vi "Fetch.vi"(8 "error in (no error)":errorcluster, 10 "Fetch Type":i32(ring) items=["CURR", "VOLT", "POW"], 11 "VISA resource name":refnum<visa-resource-name>) -> (0 "error out":errorcluster, 2 "Value":dbl, 3 "VISA resource name out":refnum<visa-resource-name>)   [LabVIEW 2020, in "IT6500.lvlib"]
doc: "<b>Valid Values:</b>\n0:Get Current\n1:Get Voltage\n2:Get Power\n\nDefault: 0:Get Current"
uses:
  IT6500.lvlib
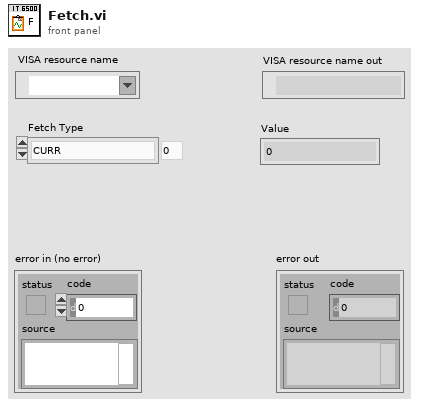
[diagram p1: front panel]
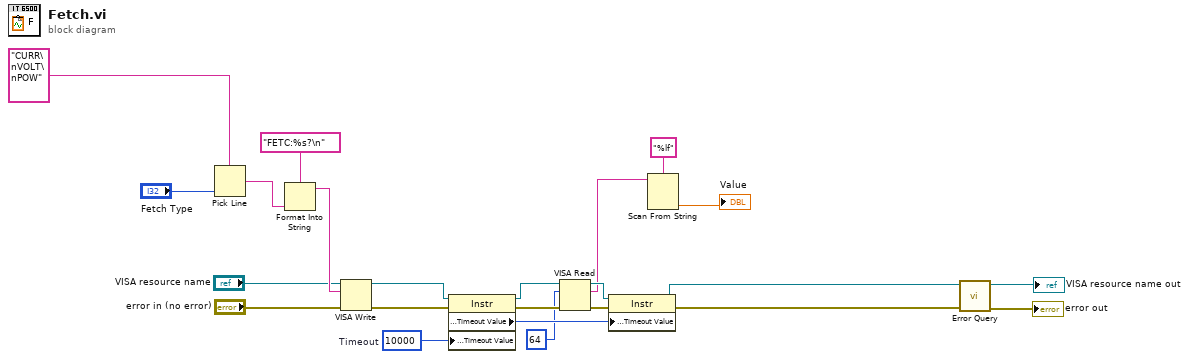
[diagram p0: block diagram]
diagram:
  w21 = u32 10000  # Timeout
  n1 = Pick Line(multi-line string="CURR\nVOLT\nPOW", line index="Fetch Type") -> (output string=w8:string)  [unwired: 1 in]
  n2 = Format Into String(format string="FETC:%s?\n", w8) -> (resulting string=w11:string)  [unwired: 2 in, 1 out]
  n3 = VISA Write(VISA resource name="VISA resource name", write buffer=w11, error in (no error)="error in (no error)") -> (VISA resource name out=w23:refnum<visa-resource-name>, error out=w22:errorcluster)  [unwired: 1 out]
  n4 = property class="Instr"(reference=w23, error in=w22, "General Settings:Timeout Value"=w21) -> (reference out=w16:refnum<visa-resource-name>, error out=w17:errorcluster, "General Settings:Timeout Value"=w18:u32)
  n5 = VISA Read(VISA resource name=w16, byte count=64, error in (no error)=w17) -> (VISA resource name out=w20:refnum<visa-resource-name>, read buffer=w13:string, error out=w19:errorcluster)  [unwired: 1 out]
  n6 = property class="Instr"(reference=w20, error in=w19, "General Settings:Timeout Value"=w18) -> (reference out=w2:refnum<visa-resource-name>, error out=w1:errorcluster)
  n7 = Scan From String(format string="%lf", input string=w13) -> (output 1=→"Value":dbl)  [unwired: 3 in, 3 out]
  n8 = call "Error Query.vi"("error in (no error)"=w1, "VISA resource name"=w2) -> ("error out"=→"error out":errorcluster, "VISA resource name out"=→"VISA resource name out":refnum<visa-resource-name>)  [unwired: 6 in, 2 out]
